vi "StringVersionToLibraryVersion.vi"(8 "error in (no error)":errorcluster, 11 "Version (as serialized)":string) -> (0 "error out":errorcluster, 2 "default data?":bool, 3 "Library Version":T1)   [LabVIEW 2019, in "BlueSerialization.lvlib" / "BlueSerializer.lvclass"]
uses:
  BlueSerializer.lvclass
  <vilib>/Utility/EditLVLibs/LibVersion.ctl
  <vilib>/regexp/Match Regular Expression.xnode
  <vilib>/Utility/EditLVLibs/Edit LVLibs.lvlib
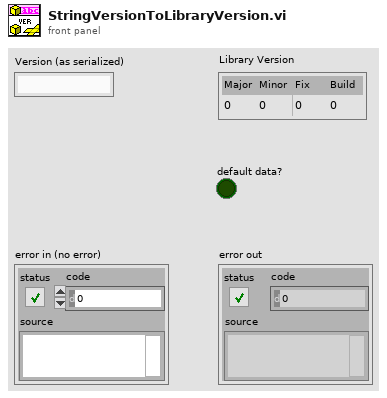
[diagram p1: front panel]
types:
  T1 = typedef "Edit LVLibs.lvlib/LibVersion.ctl" = cluster{"Major":u16, "Minor":u16, "Fix":u16, "Build":u16}
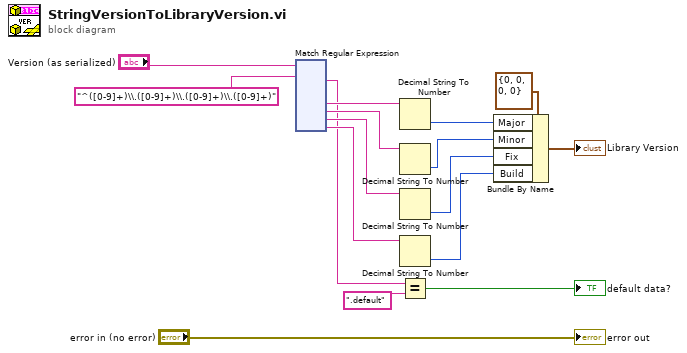
[diagram p0: block diagram]
diagram:
  n1 = xnode "Match Regular Expression"("input string"="Version (as serialized)", "regular expression"="^([0-9]+)\\.([0-9]+)\\.([0-9]+)\\.([0-9]+)") -> ("after match"=w3:string, "submatch 1"=w13:string, "submatch 2"=w11:string, "submatch 3"=w10:string, "submatch 4"=w9:string)  [unwired: 4 in, 4 out]
  n2 = Decimal String To Number(string=w13) -> (number=w12:i32)  [unwired: 2 in, 1 out]
  n3 = Decimal String To Number(string=w11) -> (number=w8:i32)  [unwired: 2 in, 1 out]
  n4 = Decimal String To Number(string=w10) -> (number=w7:i32)  [unwired: 2 in, 1 out]
  n5 = Decimal String To Number(string=w9) -> (number=w6:i32)  [unwired: 2 in, 1 out]
  n6 = Equal?(x=w3, y=".default") -> (x = y?=→"default data?":bool)
  n7 = Bundle By Name(cluster=T1 {"Major"=0, "Minor"=0, "Fix"=0, "Build"=0} ("Library Version"), "Major"=w12, "Minor"=w8, "Fix"=w7, "Build"=w6) -> (→"Library Version":T1)
  "error out" <- "error in (no error)"
